vi "SubVI.vi"(11 "% Done Ref":refnum<vi>) -> ()   [LabVIEW 2019]
panel:
  out "Numeric":i32
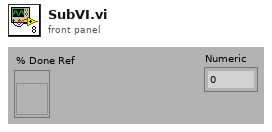
[diagram p1: front panel]
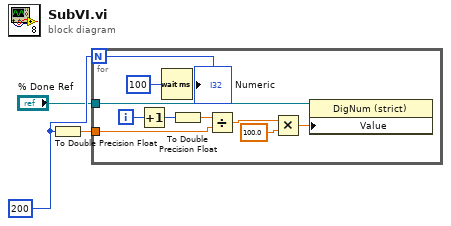
[diagram p0: block diagram]
diagram:
  w3 = 200 ("Numeric")
  n1 = To Double Precision Float(number=w3) -> (double precision float=w2:dbl)
  n2 = for {
    N: w3 -> [w4]
    tunnel: w2 -> [w12]
    tunnel: "% Done Ref" -> [w10]
    i -> [w9]
    n3 = Increment(x=w9) -> (x+1=w8:i32)
    n4 = Wait (ms)(milliseconds to wait=u32 100) -> ()  [unwired: 1 out]
    n5 = To Double Precision Float(number=w8) -> (double precision float=w11:dbl)
    n6 = Divide(x=w11, y=w12) -> (x/y=w7:dbl)
    n7 = Multiply(x=w7, y=100.0) -> (x*y=w6:dbl)
    n8 = property class="DigNum (strict)"(reference=w10, "Value"=w6) -> ()  [unwired: 1 in, 2 out]
    "Numeric" <- w4
  }
